vi "GasData.vi"(7 "file path (dialog if empty)":path, 8 "error in (no error)":errorcluster, 10 "Cluster in":T1, 11 "VISA Refnum in":refnum<visa-resource-name>) -> (0 "error out":errorcluster, 2 "ArrayINT":i64[][](array[numeric]))   [LabVIEW 2020]
uses:
  <vilib>/Utility/file.llb/Read From Spreadsheet File (I64).vi
  <vilib>/NI Modbus.llb/MB Serial Master Query Write Multiple Registers (poly).vi
  MB Serial Master Query Write Single Register (poly).vi
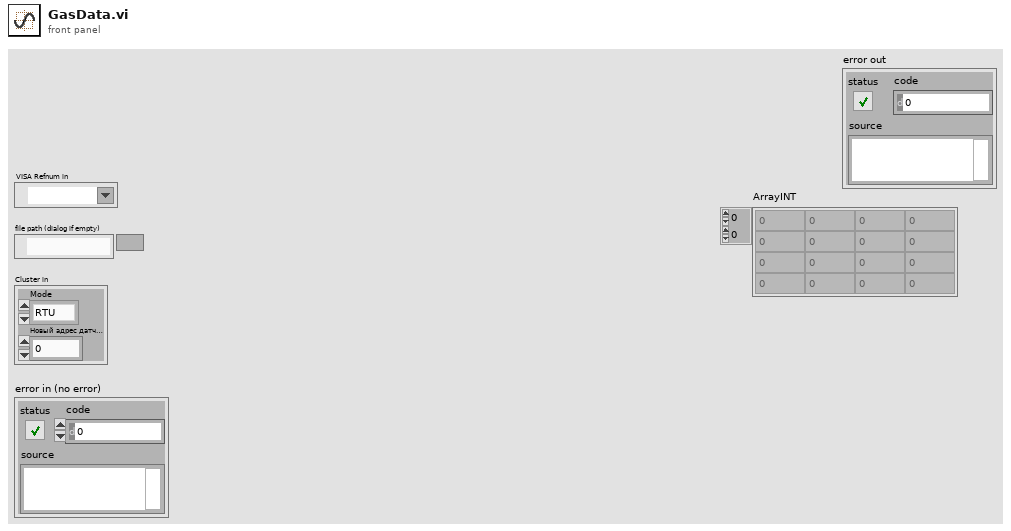
[diagram p1: front panel]
types:
  T1 = cluster{"Mode":enum16{"RTU", "ASCII"}, "Новый адрес датчика":u16}
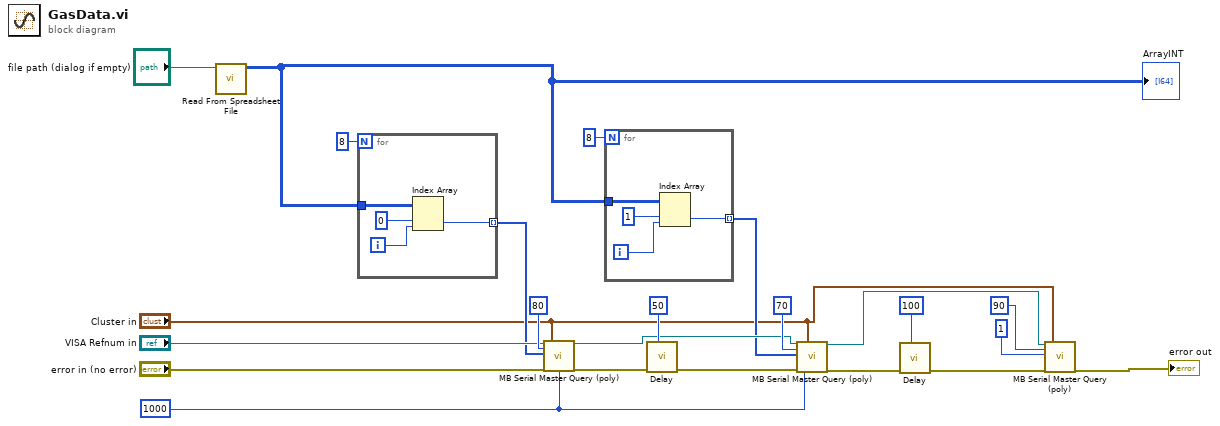
[diagram p0: block diagram]
diagram:
  w10 = u32 1000 ("Timeout")
  n1 = call-poly <vilib>:"Read From Spreadsheet File.vi"("file path (dialog if empty)"="file path (dialog if empty)") -> ("all rows"=w2:i64[][])  [unwired: 6 in, 4 out]
  "ArrayINT" <- w2
  n2 = for {
    N: 8 -> [_]
    tunnel: w2 -> [w27]
    tunnel: [w24] -> w11 mode=indexing
    i -> [w26]
    n3 = Index Array(array=w27, index (row)=0, index (col)=w26) -> (element=w24:i64)
  }
  n4 = call-poly <vilib>:"MB Serial Master Query (poly).vi"("VISA resource name"="VISA Refnum in", "Starting Address"=u16 80, "Registers"=w11, "Timeout"=w10, "error in"="error in (no error)", "Serial Parameters"="Cluster in") -> ("VISA resource name out"=w12:refnum<visa-resource-name>, "error out"=w20:errorcluster)  [unwired: 11 in, 1 out]
  n5 = for {
    N: 8 -> [_]
    tunnel: w2 -> [w31]
    tunnel: [w28] -> w9 mode=indexing
    i -> [w30]
    n6 = Index Array(array=w31, index (row)=1, index (col)=w30) -> (element=w28:i64)
  }
  n7 = call "Delay.vi"("milliseconds to wait"=u32 50, "error in (no error)"=w20) -> ("error out"=w13:errorcluster)  [unwired: 8 in, 1 out]
  n8 = call-poly <vilib>:"MB Serial Master Query (poly).vi"("VISA resource name"=w12, "Starting Address"=u16 70, "Registers"=w9, "Timeout"=w10, "error in"=w13, "Serial Parameters"="Cluster in") -> ("VISA resource name out"=w4:refnum<visa-resource-name>, "error out"=w17:errorcluster)  [unwired: 12 out]
  n9 = call "Delay.vi"("milliseconds to wait"=u32 100, "error in (no error)"=w17) -> ("error out"=w8:errorcluster)  [unwired: 8 in, 1 out]
  n10 = call-poly <vilib>:"MB Serial Master Query (poly).vi"("VISA resource name"=w4, "Address"=u16 90 ("Command"), "Holding Register"=u16 1 ("Data"), "error in"=w8, "Serial Parameters"="Cluster in") -> ("error out"=→"error out":errorcluster)  [unwired: 1 in, 13 out]
